vi "Teleop.vi"(10 "Match Info":T1={"Autonomous Elapsed Seconds"=0.0, "TeleOp Elapsed Seconds"=0.0, "Disabled Elapsed Seconds"=0.0, "Visited Autonomous"=FALSE, "Visited TeleOp"=FALSE, "Visited Disabled"=FALSE, "Autonomous Settings"={"Autonomous Style"=enum."Independent", "VI Refnum"=refnum}}, 11 "Call Context":T2) -> ()   [LabVIEW 2015]
doc: "This VI is called for each TeleOp packet received from the DS where the robot is not disabled. It is often used to read from the joysticks and update I/O or to update setpoints for timed control loops. It should complete and return within 20 milliseconds or it may miss DS packets."
uses:
  <vilib>/Rock Robotics/WPI/DriverStation/WPI_DriverStationDerivedRobotMode.ctl
  <vilib>/Rock Robotics/WPI/DriverStation/WPI_DriverStationMatch Info.ctl
  <vilib>/Rock Robotics/WPI/Utilities/WPI_GetSetVariantRefNum.vi
  <vilib>/Rock Robotics/Network Tables/NT Write Boolean Array.vi
  <vilib>/Rock Robotics/Network Tables/NT Write Numeric Array.vi
  <vilib>/Rock Robotics/Network Tables/NT Read Boolean.vi
  Robot Global Data.vi
  <vilib>/Rock Robotics/WPI/RobotDrive/WPI_RobotDriveArcadeDrive_Standard(NoSaturation).vi
  <vilib>/Rock Robotics/Network Tables/NT Read Number.vi
panel:
  out "Sample Slider 0":dbl(slide) scale=0.0..5.0
  out "Sample Boolean 1":bool
  out "Sample Boolean 0":bool
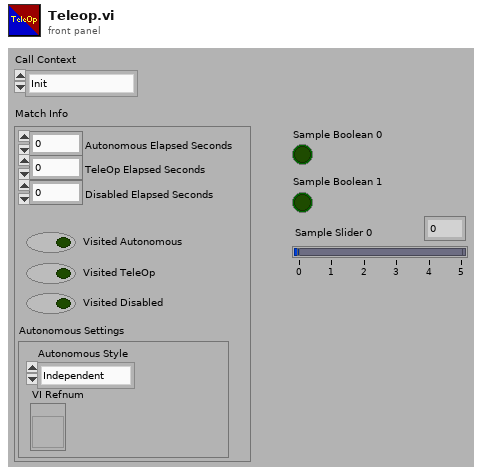
[diagram p1: front panel]
types:
  T1 = typedef "WPI_DriverStationMatch Info.ctl" = cluster{"Autonomous Elapsed Seconds":dbl, "TeleOp Elapsed Seconds":dbl, "Disabled Elapsed Seconds":dbl, "Visited Autonomous":bool, "Visited TeleOp":bool, "Visited Disabled":bool, "Autonomous Settings":cluster{"Autonomous Style":enum16{"Iterative", "Independent"}, "VI Refnum":refnum<vi>}}
  T2 = typedef "WPI_DriverStationDerivedRobotMode.ctl" = enum16{"Init", "Execute", "Stop"}
  T3 = typedef "WPI_JoystickDevRef.ctl" = cluster{"Device":T4}
  T4 = typedef "WPI_JoystickDeviceEnum.ctl" = enum16{"USB 0", "USB 1", "USB 2", "USB 3", "USB 4", "USB 5"}
  T5 = typedef "WPI_MotorControlDeviceRef.ctl" = cluster{"DeviceStatus":errorcluster, "Type":T6, "PWM":cluster{"PWM Channel":T7, "DeadBand":T8}, "CAN":cluster{"Device Number":u8, "Control Mode":T9, "Semaphore":T10, "Max Vout":dbl, "TalonSRX Control Mode":T11}, "Invert":bool}
  T6 = typedef "WPI_MotorControlType.ctl" = enum16{"PWM", "CAN", "CANTalonSRX"}
  T7 = typedef "FPGA_DIOPWMChannel.ctl" = enum8{"PWM 0", "PWM 1", "PWM 2", "PWM 3", "PWM 4", "PWM 5", "PWM 6", "PWM 7", "PWM 8", "PWM 9", "PWM MXP 0", "PWM MXP 1", "PWM MXP 2", "PWM MXP 3", "PWM MXP 4", "PWM MXP 5", "PWM MXP 6", "PWM MXP 7", "PWM MXP 8", "PWM MXP 9", "Invalid"}
  T8 = typedef "WPI_PWMDeadband.ctl" = cluster{"Name":string, "maxPositivePwm":i32, "minPositivePwm":i32, "centerPwm":i32, "maxNegativePwm":i32, "minNegativePwm":i32, "angularRange":u16}
  T9 = typedef "WPI_CANJaguar_ControlMode.ctl" = enum8{"Percent VBus", "Current", "Speed", "Position", "Voltage"}
  T10 = typedef "Semaphore RefNum" = refnum<k1>
  T11 = typedef "WPI_CANTalonSRX_APIControlMode.ctl" = enum8{"Percent VBus", "Speed", "Position", "Slave", "Unchanged / Invalid", "Voltage Compensation", "Current", "Motion Profile"}
  T12 = typedef "WPI_RobotDriveDevRef.ctl" = cluster{"DevStatus":errorcluster, "Motors[]":T5[], "Square Inputs":bool, "Max Output":dbl}
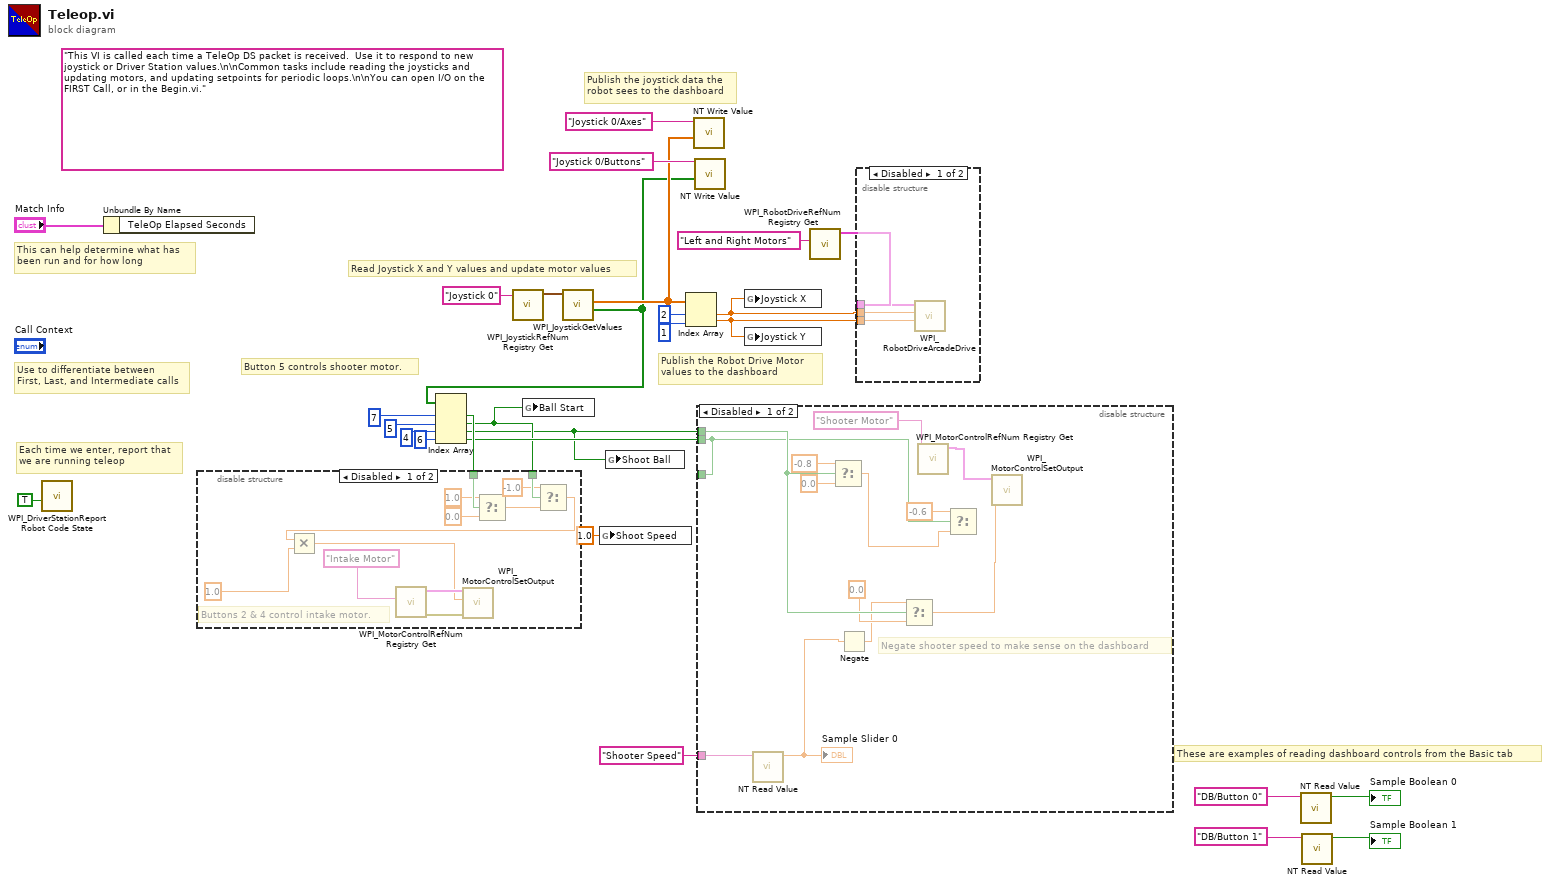
[diagram p0: block diagram]
diagram:
  (unwired) "This VI is called each time a TeleOp DS packet is received.  Use it to respond to new joystick or Driver Station values.\n\nCommon tasks include reading the joysticks and updating motors, and updating setpoints for periodic loops.\n\nYou can open I/O on the FIRST Call, or in the Begin.vi."
  # "Button 5 controls shooter motor."
  # "These are examples of reading dashboard controls from the Basic tab"
  # "Publish the Robot Drive Motor\nvalues to the dashboard"
  # "Publish the joystick data the\nrobot sees to the dashboard"
  # "Each time we enter, report that\nwe are running teleop"
  # "Use to differentiate between\nFirst, Last, and Intermediate calls"
  # "This can help determine what has\nbeen run and for how long"
  # "Read Joystick X and Y values and update motor values"
  n1 = call <vilib>:"WPI_DriverStationReport Robot Code State.vi"("TeleOp"=TRUE ("Autonomous")) -> ()  [unwired: 10 in, 1 out]
  n2 = Unbundle By Name("Match Info") -> ()  [unwired: 1 out]
  n3 = call <vilib>:"WPI_JoystickRefNum Registry Get.vi"("refnum name"="Joystick 0") -> ("JoystickDevRef"=w26:T3)  [unwired: 1 in, 9 out]
  n4 = call <vilib>:"WPI_JoystickGetValues.vi"("JoystickDevRef"=w26) -> ("Buttons"=w13:bool[], "Axes"=w22:dbl[])  [unwired: 6 in, 3 out]
  n5 = Index Array(array=w13, index #1=7 ("index"), index #2=5 ("index"), index #3=4 ("index"), index #4=6 ("index")) -> (element #1=w10:bool, element #2=w4:bool, element #3=w2:bool, element #4=w5:bool)
  n6 = disable-structure shown="Disabled" {
    disable-tunnel: w10 -> [w37 _]
    disable-tunnel: w4 -> [w34 _]
    frame Disabled {
      # "Buttons 2 & 4 control intake motor."
      n7 = call <vilib>:"WPI_MotorControlRefNum Registry Get.vi"("refnum name"="Intake Motor") -> ("error out"=w38:errorcluster, "MotorControlDevRef"=w40:T5)  [unwired: 9 in]
      n8 = Select(t=1.0, s=w37, f=0.0) -> (s? t:f=w33:dbl)
      n9 = Select(t=-1.0, s=w34, f=w33) -> (s? t:f=w31:dbl)
      n10 = Multiply(x=w31, y=1.0) -> (x*y=w30:dbl)
      n11 = call <vilib>:"WPI_MotorControlSetOutput.vi"("error in (no error)"=w38, "Output"=w30, "MotorControlDevRef"=w40) -> ()  [unwired: 6 in, 3 out]
    }
    frame Enabled {
    }
  }
  n12 = global write "Robot Global Data.vi" "Ball Start"(w4) -> ()
  n13 = global write "Robot Global Data.vi" "Shoot Speed"(1.0 ("Shoot Speed")) -> ()
  n14 = global write "Robot Global Data.vi" "Shoot Ball"(w2) -> ()
  n15 = Index Array(array=w22, index #1=2 ("index"), index #2=1 ("index")) -> (element #1=w7:dbl, element #2=w9:dbl)
  n16 = call-poly <vilib>:"NT Write Value.vi"("Numeric Array"=w22, "Name"="Joystick 0/Axes") -> ()  [unwired: 9 in, 1 out]
  n17 = call-poly <vilib>:"NT Write Value.vi"("Boolean Array"=w13, "Name"="Joystick 0/Buttons") -> ()  [unwired: 9 in, 1 out]
  n18 = disable-structure shown="Disabled" {
    disable-tunnel: "Shooter Speed" ("refnum name") -> [w53 _]
    disable-tunnel: w2 -> [w50 _]
    disable-tunnel: w5 -> [w41 _]
    disable-tunnel: [w41 _] -> _
    frame Disabled {
      # "Negate shooter speed to make sense on the dashboard"
      n19 = call-poly <vilib>:"NT Read Value.vi"("Name"=w53) -> ("Numeric"=w44:dbl)  [unwired: 9 in, 1 out]
      "Sample Slider 0" <- w44
      n20 = Select(t=-0.8, s=w50, f=0.0) -> (s? t:f=w46:dbl)
      n21 = Negate(x=w44) -> (-x=w42:dbl)
      n22 = Select(t=w42, s=w50, f=0.0) -> (s? t:f=w45:dbl)
      n23 = call <vilib>:"WPI_MotorControlRefNum Registry Get.vi"("refnum name"="Shooter Motor") -> ("MotorControlDevRef"=w51:T5)  [unwired: 9 in, 1 out]
      n24 = Select(t=-0.6, s=w41, f=w46) -> ()  [unwired: 1 out]
      n25 = call <vilib>:"WPI_MotorControlSetOutput.vi"("Output"=w45, "MotorControlDevRef"=w51) -> ()  [unwired: 7 in, 3 out]
    }
    frame Enabled {
    }
  }
  n26 = global write "Robot Global Data.vi" "Joystick X"(w7) -> ()
  n27 = global write "Robot Global Data.vi" "Joystick Y"(w9) -> ()
  n28 = call <vilib>:"WPI_RobotDriveRefNum Registry Get.vi"("refnum name"="Left and Right Motors") -> ("RobotDriveDevRef"=w15:T12)  [unwired: 9 in, 1 out]
  n29 = disable-structure shown="Disabled" {
    disable-tunnel: w7 -> [w56 _]
    disable-tunnel: w9 -> [w55 _]
    disable-tunnel: w15 -> [w54 _]
    frame Disabled {
      n30 = call-poly <vilib>:"WPI_RobotDriveArcadeDrive.vi"("Y axis value"=w55, "X axis value"=w56, "RobotDriveDevRef"=w54) -> ()  [unwired: 6 in, 3 out]
    }
    frame Enabled {
    }
  }
  n31 = call-poly <vilib>:"NT Read Value.vi"("Name"="DB/Button 0" ("refnum name")) -> ("Boolean"=→"Sample Boolean 0":bool)  [unwired: 9 in, 1 out]
  n32 = call-poly <vilib>:"NT Read Value.vi"("Name"="DB/Button 1" ("refnum name")) -> ("Boolean"=→"Sample Boolean 1":bool)  [unwired: 9 in, 1 out]
